vi "Update Test Plan.vi"(8 "error in (no error)":errorcluster, 10 "Status":string="PENDING_APPROVAL", 11 "Test Plan ID":string="1215195") -> (0 "error out":errorcluster)   [LabVIEW 2024]
uses:
  <vilib>/Skyline/Configuration/Configuration HTTP_class/NI Skyline Configuration HTTP.lvclass/NI Skyline Configuration HTTP.ctl
  <vilib>/Skyline/Configuration/Configuration HTTP_class/Read Server URL.vi
  <vilib>/Skyline/Configuration/Configuration HTTP_class/Open Configuration HTTP Auto.vi
  <vilib>/httpClient/POSTBuffer.vi
  <vilib>/Skyline/Configuration/Configuration HTTP_class/NI Skyline Configuration HTTP.lvclass
  <vilib>/httpClient/LabVIEWHTTPClient.lvlib
panel:
  out "body":string
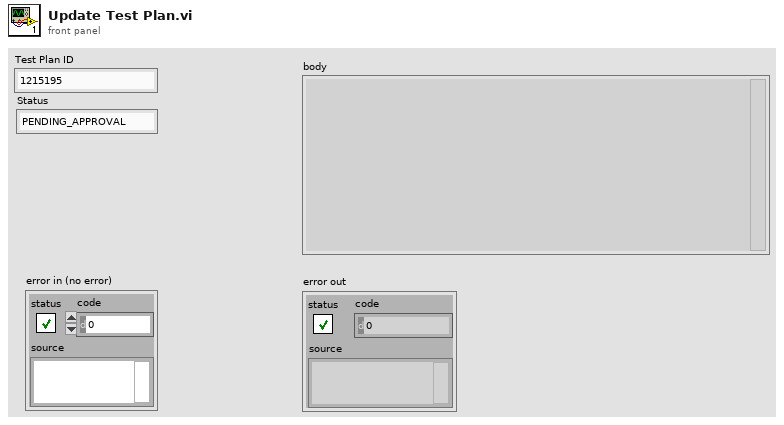
[diagram p1: front panel]
types:
  T1 = typedef "LabVIEWHTTPClient.lvlib/ClientHandle.ctl" = refnum<k1>
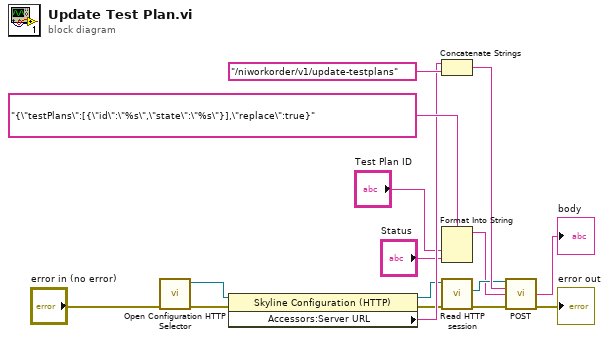
[diagram p0: block diagram]
diagram:
  n1 = call-poly <vilib>:"Open Configuration HTTP Selector.vi"("error in (no error)"="error in (no error)") -> ("error out"=w9:errorcluster, "configuration"=w7:refnum<class "NI Skyline Configuration HTTP.lvclass">)  [unwired: 9 in]
  n2 = property on="Property Node" class="Skyline Configuration (HTTP)"(reference=w7, error in=w9) -> (reference out=w12:refnum<class "NI Skyline Configuration HTTP.lvclass">, error out=w8:errorcluster, "Accessors:Server URL"=w13:string)
  n3 = Concatenate Strings(w13, "/niworkorder/v1/update-testplans" ("url")) -> (w15:string)
  n4 = Format Into String(format string="{\"testPlans\":[{\"id\":\"%s\",\"state\":\"%s\"}],\"replace\":true}", "Test Plan ID", "Status") -> (resulting string=w2:string)  [unwired: 2 in, 1 out]
  n5 = call <vilib>:"Read HTTP session.vi"("error in (no error)"=w8, "HTTP configuration in"=w12) -> ("error out"=w11:errorcluster, "http session"=w10:T1)  [unwired: 7 in, 1 out]
  n6 = call-poly <vilib>:"POST.vi"("client handle"=w10, "url"=w15, "buffer"=w2, "error in (no error)"=w11) -> ("body"=→"body":string, "error out"=→"error out":errorcluster)  [unwired: 8 in, 2 out]
